vi "subMFD_FXP Modeling & Simu.vi"() -> ()   [LabVIEW 2023]
uses:
  <vilib>/addons/Digital Filter Design/_Objects.llb/DFD Multirate Filter Obj.ctl
  <vilib>/addons/Digital Filter Design/_Objects.llb/DFD Multirate Mode.ctl
  <vilib>/addons/Digital Filter Design/_Objects.llb/DFD Coef Norm Type.ctl
  <vilib>/addons/Digital Filter Design/_Objects.llb/DFD Round-off Mode.ctl
  <vilib>/addons/Digital Filter Design/_Objects.llb/DFD FXP MRate Multiply Mode.ctl
  <vilib>/addons/Digital Filter Design/_Objects.llb/DFD Quantization Settings.ctl
  <vilib>/addons/Digital Filter Design/_Objects.llb/DFD Quantization Sources.ctl
  <vilib>/addons/Digital Filter Design/FXPMRateSim.llb/DFD FXP MRate Simulation (DBL).vi
  <vilib>/addons/Digital Filter Design/Multirate.llb/DFD MRate Filtering (Array).vi
  <vilib>/addons/Digital Filter Design/FilterLib.llb/DFD Save MRate Filter to File.vi
  <vilib>/Analysis/NI_AALBase.lvlib
  <vilib>/Analysis/NI_AALPro.lvlib
  <vilib>/addons/Digital Filter Design/NI_DigFilterLicensed.lvlib
panel:
  in  "Amplitude":dbl=0.5 min=0.001 max=1.0 step=0.001
  in  "Random Input":bool
  in  "Frequency":dbl=1000.1 max=0.5 format="%#_4p Hz"
  in  "Pure Sine Input":bool=TRUE
  in  "Output Rounding Mode":u16(ring)=1 items=["Nearest", "Truncation"]
  in  "Output Word Length":i16=16 min=1 max=32 step=1
  in  "Input Word Length":i16=16 min=1 max=32 step=1
  in  "Save Multirate Filter to File":bool
  in  "Run":bool
  out "MSE":dbl format="%.3e"
  out "Simulation Results":dbl[][](graph)
  out "Successful Design?":bool
  out "multirate filter out":T1={"mMRate_Structure"=enum."FIR", "mMRate_Mode"=0, "mMRate_Factor"=-1, "mMRate_FIRParams"={"mMRate_FIR_H"=[], "mMRate_FIR_IsNyquist?"=FALSE, "mMRate_FIR_IsSymmetric?"=FALSE}, "mMRate_CICParams"={"mMRate_CIC_#Stage"=0, "mMRate_CIC_Lag"=1, "mMRate_CIC_Type"=enum."Lowpass"}, "mMRate_Order"=0, "mMRate_Version"="2.0", "mMRate_Comments"="", "mMRate_RationalFactor"={"mMRate_L"=-1, "mMRate_M"=-1}, "mMRate_Fs"=1.0, "mMRate_Quantized?"=FALSE, "mMRate_QFilterGain"=1.0, "mMRate_CoefWl"=16, "mMRate_Scaling"={"mMRate_ScaleByPowerOf2?"=FALSE, "mMRate_ScaleType"=enum."No Norm"}, "mMRate_InputWl"=16, "mMRate_OutputWl"=16, "mMRate_OutputMode"=enum."Truncation", "mMRate_MultMode"=enum."Truncated", "mMRate_BitPruning"=FALSE, "mMRate_GainWl"=16, "mMRate_OutputFwl"=0, "mMRate_SumIwl"=0, "mMRate_InputIwl "=16, "mMRate_SumWl"=32, "mMRate_CoefIwl"=0} {"mMRate_SumWl" min=1 max=32 step=1; "mMRate_InputIwl" min=1 max=32 step=1; "mMRate_GainWl" min=1 max=32 step=1; "mMRate_OutputWl" min=1 max=32 step=1; "mMRate_InputWl" min=1 max=32 step=1; "mMRate_CoefWl" min=1 max=32 step=1; "mMRate_Mode" items=["Default"=-1, "No Rate Change"=0, "Interpolation"=1, "Decimation"=2, "Interpolated"=3, "Rational"=4]}
  in  "multirate filter in":T1={"mMRate_Structure"=enum."FIR", "mMRate_Mode"=0, "mMRate_Factor"=-1, "mMRate_FIRParams"={"mMRate_FIR_H"=[], "mMRate_FIR_IsNyquist?"=FALSE, "mMRate_FIR_IsSymmetric?"=FALSE}, "mMRate_CICParams"={"mMRate_CIC_#Stage"=0, "mMRate_CIC_Lag"=1, "mMRate_CIC_Type"=enum."Lowpass"}, "mMRate_Order"=0, "mMRate_Version"="2.0", "mMRate_Comments"="", "mMRate_RationalFactor"={"mMRate_L"=-1, "mMRate_M"=-1}, "mMRate_Fs"=1.0, "mMRate_Quantized?"=FALSE, "mMRate_QFilterGain"=1.0, "mMRate_CoefWl"=16, "mMRate_Scaling"={"mMRate_ScaleByPowerOf2?"=FALSE, "mMRate_ScaleType"=enum."No Norm"}, "mMRate_InputWl"=16, "mMRate_OutputWl"=16, "mMRate_OutputMode"=enum."Truncation", "mMRate_MultMode"=enum."Truncated", "mMRate_BitPruning"=FALSE, "mMRate_GainWl"=16, "mMRate_OutputFwl"=0, "mMRate_SumIwl"=0, "mMRate_InputIwl "=16, "mMRate_SumWl"=32, "mMRate_CoefIwl"=0} {"mMRate_SumWl" min=1 max=32 step=1; "mMRate_InputIwl" min=1 max=32 step=1; "mMRate_GainWl" min=1 max=32 step=1; "mMRate_OutputWl" min=1 max=32 step=1; "mMRate_InputWl" min=1 max=32 step=1; "mMRate_CoefWl" min=1 max=32 step=1; "mMRate_Mode" items=["Default"=-1, "No Rate Change"=0, "Interpolation"=1, "Decimation"=2, "Interpolated"=3, "Rational"=4]}
  out "OK":bool
  in  "stop":bool
  # "Simulation Results"
  # "Fixed-Point Filter Modeling"
  # "Input \nWord Length"
  # "MSE"
  # "Output \nWord Length"
  # "Output \nRounding Mode"
  # "Simulation Source"
  # "Frequency"
  # "Amplitude"
  # "Demo Program"
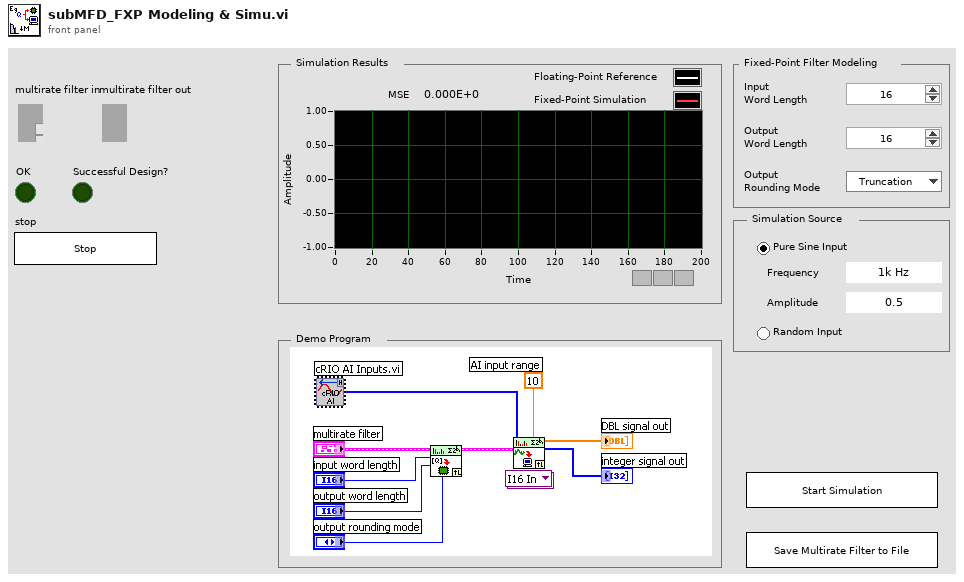
[diagram p1: front panel]
types:
  T1 = typedef "NI_DigFilterLicensed.lvlib/DFD Multirate Filter Obj.ctl" = cluster{"mMRate_Structure":enum16{"CIC", "FIR", "IIR", "Lattice"}, "mMRate_Mode":T2, "mMRate_Factor":i32, "mMRate_FIRParams":cluster{"mMRate_FIR_H":dbl[], "mMRate_FIR_IsNyquist?":bool, "mMRate_FIR_IsSymmetric?":bool}, "mMRate_CICParams":cluster{"mMRate_CIC_#Stage":i32, "mMRate_CIC_Lag":i32, "mMRate_CIC_Type":enum16{"Lowpass", "Highpass"}}, "mMRate_Order":i32, "mMRate_Version":string, "mMRate_Comments":string, "mMRate_RationalFactor":cluster{"mMRate_L":i32, "mMRate_M":i32}, "mMRate_Fs":dbl, "mMRate_Quantized?":bool, "mMRate_QFilterGain":dbl, "mMRate_CoefWl":i16, "mMRate_Scaling":cluster{"mMRate_ScaleByPowerOf2?":bool, "mMRate_ScaleType":T3}, "mMRate_InputWl":i16, "mMRate_OutputWl":i16, "mMRate_OutputMode":T4, "mMRate_MultMode":T5, "mMRate_BitPruning":bool, "mMRate_GainWl":i16, "mMRate_OutputFwl":i16, "mMRate_SumIwl":i16, "mMRate_InputIwl ":i16, "mMRate_SumWl":i16, "mMRate_CoefIwl":i16}
  T2 = typedef "NI_DigFilterLicensed.lvlib/DFD Multirate Mode.ctl" = i16
  T3 = typedef "NI_DigFilterLicensed.lvlib/DFD Coef Norm Type.ctl" = enum16{"No Norm", "Time Domain 1-Norm", "Time Domain 2-Norm", "Time Domain Inf-Norm"}
  T4 = typedef "NI_DigFilterLicensed.lvlib/DFD Round-off Mode.ctl" = enum16{"Nearest", "Truncation"}
  T5 = typedef "NI_DigFilterLicensed.lvlib/DFD FXP MRate Multiply Mode.ctl" = enum16{"Truncated", "Full"}
  T6 = typedef "NI_DigFilterLicensed.lvlib/DFD Quantization Settings.ctl" = cluster{"source":T7, "wl":i16, "iwl":i16, "overflow mode":enum16{"Saturation", "Wrap"}, "rounding mode":enum16{"Nearest", "Truncation"}, "signed?":bool}
  T7 = typedef "NI_DigFilterLicensed.lvlib/DFD Quantization Sources.ctl" = u16
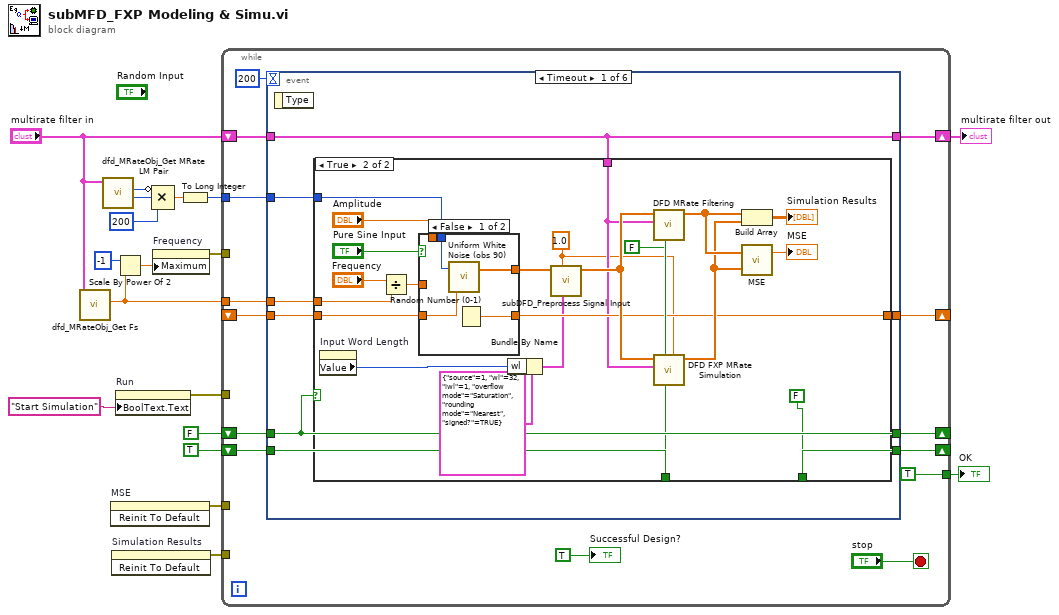
[diagram p0: block diagram]
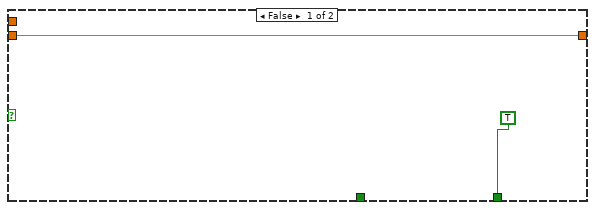
[diagram p2: hidden frame]
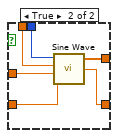
[diagram p3: hidden frame]
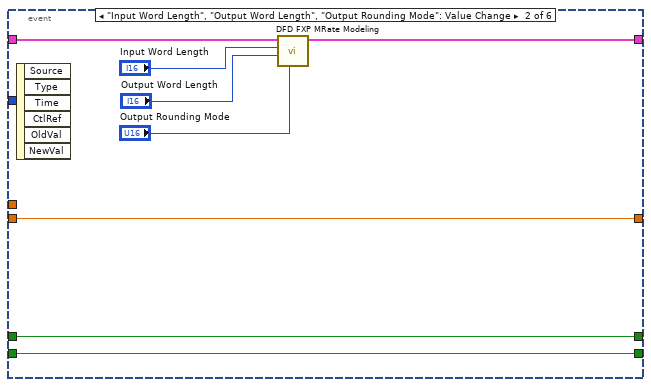
[diagram p4: hidden frame]
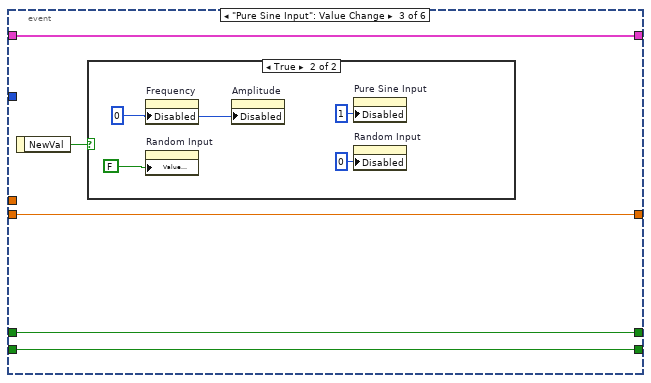
[diagram p5: hidden frame]
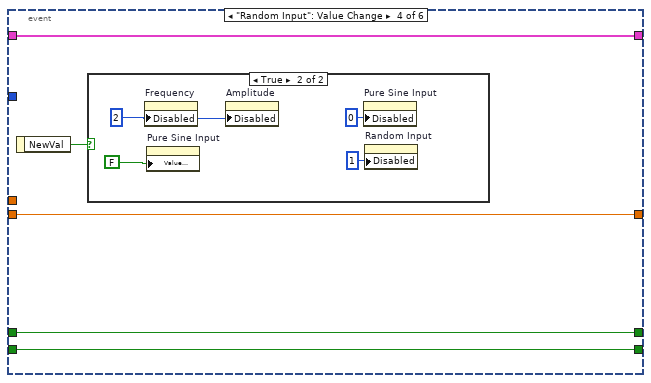
[diagram p7: hidden frame]
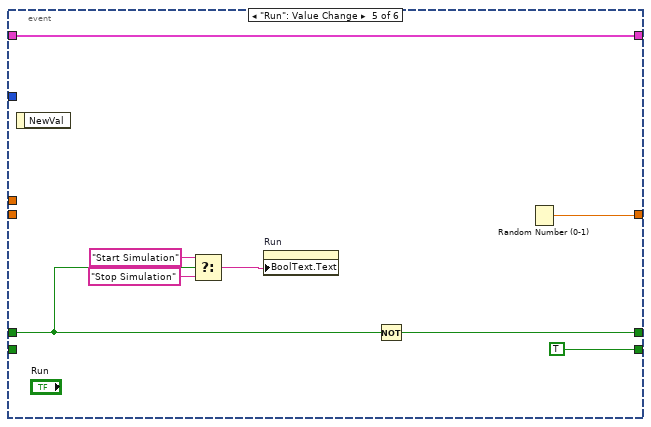
[diagram p9: hidden frame]
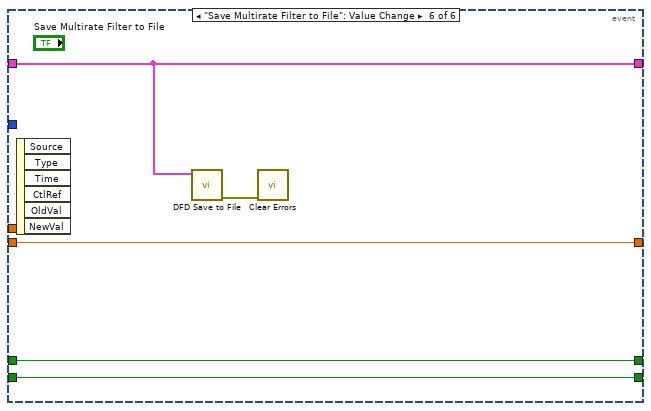
[diagram p10: hidden frame]
diagram:
  n1 = call <vilib>:"dfd_MRateObj_Get Fs.vi"("multirate filter in"="multirate filter in") -> ("fs"=w5:dbl)  [unwired: 10 out]
  n2 = call <vilib>:"dfd_MRateObj_Get MRate LM Pair.vi"("multirate filter in"="multirate filter in") -> ("M"=w9:i32, "L"=w10:i32)  [unwired: 1 in, 8 out]
  n3 = invoke on="MSE" class="DigNum (strict)" method="Reinit To Default"() -> (error out=w15:errorcluster)  [unwired: 3 in, 2 out]
  n4 = invoke on="Simulation Results" class="WFGraph (strict)" method="Reinit To Default"() -> (error out=w14:errorcluster)  [unwired: 3 in, 2 out]
  n5 = Scale By Power Of 2(n=-1, x=w5) -> (x*2^n=w7:dbl)
  n6 = property on="Run" class="Bool"("BoolText.Text"="Start Simulation" ("t")) -> (error out=w13:errorcluster)  [unwired: 2 in, 1 out]
  n7 = Compound Arithmetic op=MULTIPLY(invert w10, w9, 200 ("value")) -> (w3:dbl)
  n8 = property on="Frequency" class="DigNum (strict)"("Maximum"=w7) -> (error out=w4:errorcluster)  [unwired: 2 in, 1 out]
  n9 = To Long Integer(number=w3) -> (32bit integer=w2:i32)
  n10 = while {
    tunnel: [TRUE] -> w18
    shift-right: [w28] -> w17
    shift-left: "multirate filter in" -> [w29]
    shift-right: [w25] -> _
    shift-left: FALSE -> [w26]
    tunnel: w15 -> [_]
    tunnel: w14 -> [_]
    tunnel: w13 -> [_]
    shift-right: [w24] -> _
    shift-left: _ -> [w23]
    shift-right: [w22] -> _
    shift-left: TRUE -> [w21]
    tunnel: w5 -> [w20]
    tunnel: w4 -> [_]
    tunnel: w2 -> [w19]
    stop <- "stop" stop-if-true
    n11 = event shown="[0] Timeout" {
      selector: _ -> [_ _ _ _ _ _]
      dyn-events: _ -> [_ _ _ _ _ _]
      timeout: 200 -> [_ _ _ _ _ _]
      tunnel: w29 -> [w38 w82 w86 w95 w108 w113]
      tunnel: [w38 w78 w86 w95 w108 w113] -> w28
      tunnel: w26 -> [w40 w81 w85 w94 w106 w111]
      tunnel: [w40 w81 w85 w94 w107 w111] -> w25
      tunnel: w21 -> [w39 w79 w83 w92 _ w110]
      tunnel: [w37 w79 w83 w92 TRUE w110] -> w22
      tunnel: [w36 w80 w84 w93 w102 w109] -> w24
      tunnel: w23 -> [w35 w80 w84 w93 _ w109]
      tunnel: w20 -> [w34 _ _ _ _ _]
      tunnel: w19 -> [w33 _ _ _ _ _]
      event Timeout {
        n12 = event-data() -> ()  [unwired: 2 out]
        n13 = case shown="True" w40 {
          tunnel: w39 -> [_ w55]
          tunnel: w38 -> [_ w48]
          tunnel: [TRUE FALSE] -> w37
          tunnel: [w41 w53] -> w36
          tunnel: w35 -> [w41 w52]
          tunnel: w34 -> [_ w47]
          tunnel: w33 -> [_ w46]
          frame False {
          }
          frame True {
            w43 = 1.0 ("amp")
            n14 = property on="Input Word Length" class="DigNum (strict)"() -> ("Value"=w49:i16)  [unwired: 2 in, 2 out]
            n15 = Divide(x="Frequency", y=w47) -> (x/y=w62:dbl)
            n16 = case shown="False" "Pure Sine Input" {
              tunnel: w62 -> [_ w74]
              tunnel: [w68 w73] -> w58
              tunnel: [w66 w72] -> w53
              tunnel: w52 -> [w67 w71]
              tunnel: w46 -> [w65 w70]
              tunnel: "Amplitude" -> [_ w69]
              frame False {
                n17 = call <vilib>:"Uniform White Noise (obs 90).vi"("seed"=w67, "samples"=w65) -> ("uniform white noise"=w68:dbl[])  [unwired: 1 in, 1 out]
                n18 = Random Number (0-1)() -> (number: 0 to 1=w66:dbl)
              }
              frame True {
                n19 = call <vilib>:"Sine Wave.vi"("samples"=w70, "amplitude"=w69, "frequency"=w74, "phase in"=w71) -> ("sine wave"=w73:dbl[], "phase out"=w72:dbl)  [unwired: 1 in, 1 out]
              }
            }
            n20 = Bundle By Name(cluster=T6 {"source"=1, "wl"=32, "iwl"=1, "overflow mode"=enum."Saturation", "rounding mode"=enum."Nearest", "signed?"=TRUE} ("input quantizer"), "wl"=w49) -> (w50:T6)
            n21 = call <vilib>:"subDFD_Preprocess Signal Input.vi"("input quantizer"=w50, "input range"=w43, "x"=w58) -> ("q[x]"=w57:dbl[])  [unwired: 8 out]
            n22 = call-poly <vilib>:"DFD MRate Filtering.vi"("zero phase? (T)"=FALSE, "init? (F)"=w55, "multirate filter"=w48, "signal in"=w57) -> ("signal out"=w60:dbl[])  [unwired: 1 in, 6 out]
            n23 = call-poly <vilib>:"DFD FXP MRate Simulation.vi"("input range"=w43, "init? (T)"=w55, "multirate filter"=w48, "signal in"=w57) -> ("DBL signal out"=w56:dbl[])  [unwired: 1 in, 6 out]
            n24 = Build Array(w60, w56) -> (→"Simulation Results":dbl[][])
            n25 = call <vilib>:"MSE.vi"("X Values"=w56, "Y Values"=w60) -> ("mse"=→"MSE":dbl)  [unwired: 1 out]
          }
        }
      }
      event "Input Word Length", "Output Word Length", "Output Rounding Mode": Value Change {
        n26 = event-data() -> ()  [unwired: 7 out]
        n27 = call <vilib>:"DFD FXP MRate Modeling.vi"("output rounding mode"="Output Rounding Mode", "output word length"="Output Word Length", "input word length"="Input Word Length", "multirate filter in"=w82) -> ("multirate filter out"=w78:T1)  [unwired: 4 in, 3 out]
      }
      event "Pure Sine Input": Value Change {
        n28 = event-data() -> ("NewVal"=w87:bool)  [unwired: 1 out]
        n29 = case shown="True" w87 {
          frame False {
          }
          frame True {
            w88 = u8 0 ("Disabled")
            n30 = property on="Frequency" class="DigNum (strict)"("Disabled"=w88) -> ()  [unwired: 2 in, 2 out]
            n31 = property on="Random Input" class="Bool (strict)"("Value (Signaling)"=FALSE) -> ()  [unwired: 2 in, 2 out]
            n32 = property on="Amplitude" class="DigNum (strict)"("Disabled"=w88) -> ()  [unwired: 2 in, 2 out]
            n33 = property on="Pure Sine Input" class="Bool (strict)"("Disabled"=u8 1) -> ()  [unwired: 2 in, 2 out]
            n34 = property on="Random Input" class="Bool (strict)"("Disabled"=u8 0) -> ()  [unwired: 2 in, 2 out]
          }
        }
      }
      event "Random Input": Value Change {
        n35 = event-data() -> ("NewVal"=w96:bool)  [unwired: 1 out]
        n36 = case shown="True" w96 {
          frame False {
          }
          frame True {
            w97 = u8 2 ("Disabled")
            n37 = property on="Frequency" class="DigNum (strict)"("Disabled"=w97) -> ()  [unwired: 2 in, 2 out]
            n38 = property on="Pure Sine Input" class="Bool (strict)"("Value (Signaling)"=FALSE) -> ()  [unwired: 2 in, 2 out]
            n39 = property on="Amplitude" class="DigNum (strict)"("Disabled"=w97) -> ()  [unwired: 2 in, 2 out]
            n40 = property on="Pure Sine Input" class="Bool (strict)"("Disabled"=u8 0) -> ()  [unwired: 2 in, 2 out]
            n41 = property on="Random Input" class="Bool (strict)"("Disabled"=u8 1) -> ()  [unwired: 2 in, 2 out]
          }
        }
      }
      event "Run": Value Change {
        n42 = event-data() -> ()  [unwired: 2 out]
        n43 = Select(t="Start Simulation", s=w106, f="Stop Simulation") -> (s? t:f=w103:string)
        n44 = property on="Run" class="Bool"("BoolText.Text"=w103) -> ()  [unwired: 2 in, 2 out]
        n45 = Not(x=w106) -> (.not. x?=w107:bool)
        n46 = Random Number (0-1)() -> (number: 0 to 1=w102:dbl)
      }
      event "Save Multirate Filter to File": Value Change {
        n47 = event-data() -> ()  [unwired: 7 out]
        n48 = call-poly <vilib>:"DFD Save to File.vi"("multirate filter in"=w113) -> ("error out"=w112:errorcluster)  [unwired: 3 in, 7 out]
        n49 = call <vilib>:"Clear Errors.vi"("error in (no error)"=w112) -> ()  [unwired: 1 in, 6 out]
      }
    }
    "Successful Design?" <- TRUE ("Successful Design?")
  }
  "OK" <- w18
  "multirate filter out" <- w17
